vi "shutdown.vi"(11 "input cluster":T1) -> ()   [LabVIEW 2025]
uses:
  Classes/hardware/hardware.lvclass
  Classes/controller/controller.lvclass
  Classes/data log/data log.lvclass
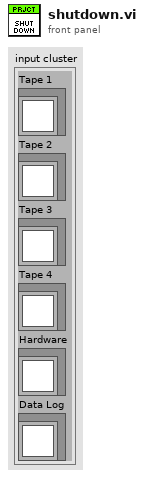
[diagram p1: front panel]
types:
  T1 = cluster{"Tape 1":refnum<class "controller.lvclass">, "Tape 2":refnum<class "controller.lvclass">, "Tape 3":refnum<class "controller.lvclass">, "Tape 4":refnum<class "controller.lvclass">, "Hardware":refnum<class "hardware.lvclass">, "Data Log":refnum<class "data log.lvclass">}
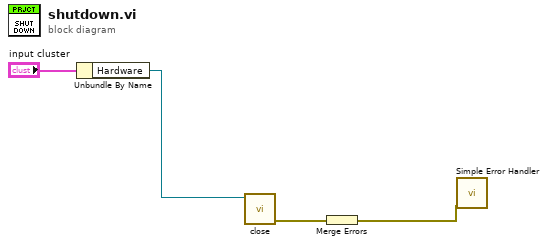
[diagram p0: block diagram]
diagram:
  n1 = Unbundle By Name("input cluster") -> ("Hardware"=w3:refnum<class "hardware.lvclass">)
  n2 = call-dynamic "close.vi"("hardware in"=w3) -> ("error out"=w2:errorcluster)  [unwired: 9 in, 1 out]
  n3 = Merge Errors(w2) -> (w1:errorcluster)
  n4 = call <vilib>:"Simple Error Handler.vi"("error in (no error)"=w1) -> ()  [unwired: 4 in, 5 out]
